vi "ADC_clean_buffer.vi"(0 "error out 2":errorcluster, 1 "task out 2":refnum<k21>) -> (2 "error out":errorcluster, 4 "task out":refnum<k21>)   [LabVIEW 2013]
uses:
  <vilib>/DAQmx/read.llb/DAQmx Read (Analog 2D DBL NChan NSamp).vi
  <vilib>/DAQmx/miscellaneous.llb/DAQmx Fill In Error Info.vi
  <resource>/objmgr/daqmx.rc
panel:
  out "data":dbl[][](array[numeric]) format="%0.2f"
  out "CurrReadPos 2":dbl
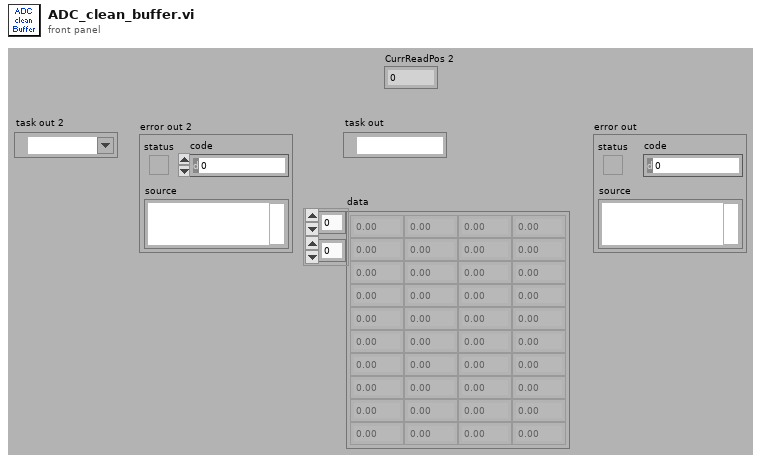
[diagram p1: front panel]
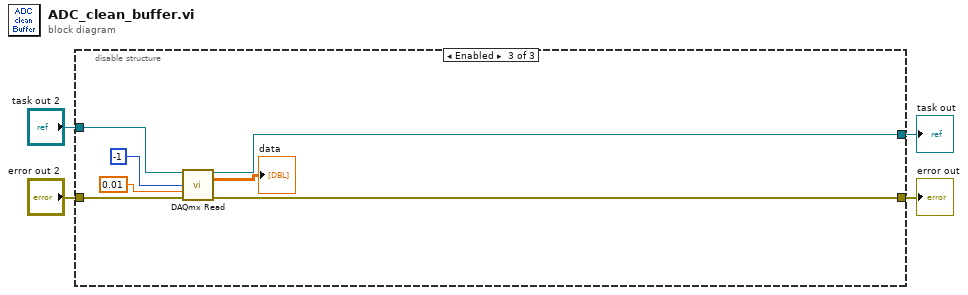
[diagram p0: block diagram]
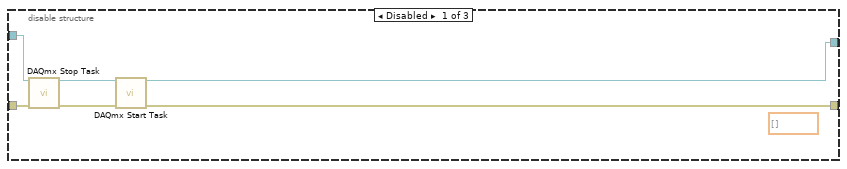
[diagram p2: hidden frame]
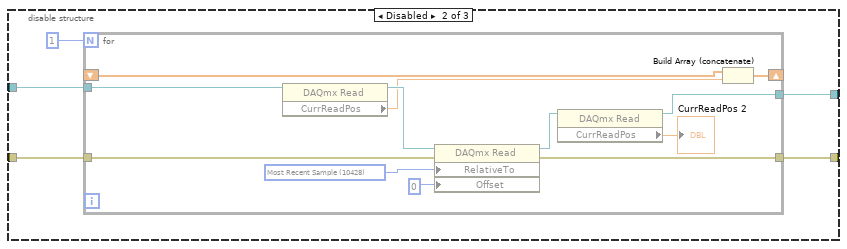
[diagram p3: hidden frame]
diagram:
  n1 = disable-structure shown="Enabled" {
    disable-tunnel: "error out 2" -> [w10 w14 w33]
    disable-tunnel: [w9 w12 w32] -> w2
    disable-tunnel: "task out 2" -> [w8 w13 w34]
    disable-tunnel: [w5 w15 w31] -> w1
    frame Disabled {
      (unwired) dbl[] [] ("Array")
      n2 = call <vilib>:"DAQmx Stop Task.vi"("task/channels in"=w8, "error in"=w10) -> ("task out"=w6:refnum<k21>, "error out"=w7:errorcluster)  [unwired: 12 in]
      n3 = call <vilib>:"DAQmx Start Task.vi"("task/channels in"=w6, "error in"=w7) -> ("task out"=w9:refnum<k21>, "error out"=w5:errorcluster)  [unwired: 12 in]
    }
    frame Disabled {
      n4 = for {
        N: 1 -> [_]
        tunnel: [w25] -> w15
        tunnel: w14 -> [w24]
        tunnel: w13 -> [w23]
        tunnel: [w20] -> w12
        shift-right: [w16] -> _
        shift-left: _ -> [w17]
        w27 = 10428 items=["First Sample"=10424, "Current Read Position"=10425, "Reference Trigger"=10426, "First Pretrigger Sample"=10427, "Most Recent Sample"=10428] ("RelativeTo")
        n5 = property class="DAQmx Read"(reference=w23) -> (reference out=w22:refnum<k21>, "CurrReadPos"=w18:dbl)  [unwired: 1 in, 1 out]
        n6 = property class="DAQmx Read"(reference=w22, error in=w24, "RelativeTo"=w27, "Offset"=0) -> (reference out=w21:refnum<k21>, error out=w25:errorcluster)
        n7 = property class="DAQmx Read"(reference=w21) -> (reference out=w20:refnum<k21>, "CurrReadPos"=→"CurrReadPos 2":dbl)  [unwired: 1 in, 1 out]
        n8 = Build Array (concatenate)(w17, w18) -> (w16:dbl[])
      }
    }
    frame Enabled {
      n9 = call-poly <vilib>:"DAQmx Read.vi"("task/channels in"=w34, "number of samples per channel"=-1, "timeout"=0.01, "error in"=w33) -> ("task out"=w32:refnum<k21>, "data"=→"data":dbl[][], "error out"=w31:errorcluster)  [unwired: 9 in]
    }
  }
  "task out" <- w2
  "error out" <- w1
